vi "New Event Handler.vi"() -> ()   [LabVIEW 2010]
doc: "이 LLB에서 이 VI를 Old Event Handler.vi와 비교합니다. 이 VI는 폴링을 사용하는 대신 이벤트 구조를 사용하여 이벤트를 처리하는 방식을 결정합니다. 변환이 다른 케이스사이에서 동작하고 다른 이벤트사이에서 전달되는 데이터를 관리하는데 하나의 시프트 레지스터만을 사용하는 경우를 이해하는 것이 더 쉽습니다. 버튼을 클릭할 때를 결정하기 위해 사용자 인터페이스를 폴링하지 않습니다. 대신에 버튼을 클릭하거나 값 변경이 발생하기를 기다리고 발생한 이벤트에 따라 무슨 일을 수행할지 결정합니다.\n\n\"데이터 수집\":\n이 버튼을 클릭하면 데이터를 수집하는 케이스를 실행합니다. \n\n\"데이터 분석 및 제시\":\n이 버튼을 클릭하면 이전에 수집한 데이터를 분석합니다. 이 버튼을 클릭하기 전에는 어떤 데이터도 수집할 필요가 없습니다. 그러나 NULL 데이터셋에 대해 수행한 분석은 어떤 유용한 정보도 제공하지 않습니다.\n\n\"정지\":\n이 버튼을 클릭하면 VI 실행을 정지합니다."
panel:
  in  "새 버튼":bool
  in  "시간 웨이브폼":waveform(dbl)={"t0"=timestamp(0 s since 1904-01-01), "dt"=0.0, "Y"=[]}
  in  "정지":bool
  in  "분석":bool
  in  "수집":bool
  # "이 VI를 실행한 후, 버튼을 눌러 해당\n이벤트를 활성화하십시오. 완료시 정지 버튼을 누르십시오."
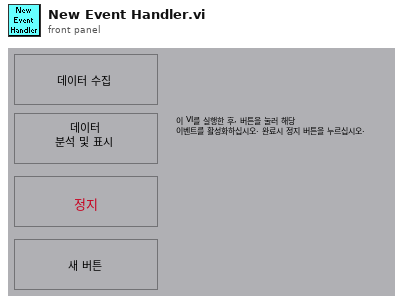
[diagram p1: front panel]
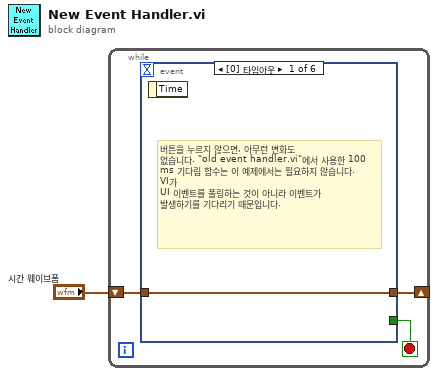
[diagram p0: block diagram]
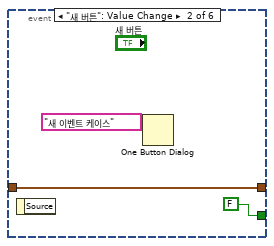
[diagram p2: hidden frame]
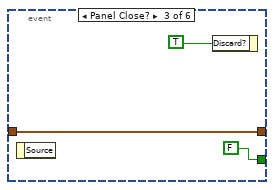
[diagram p3: hidden frame]
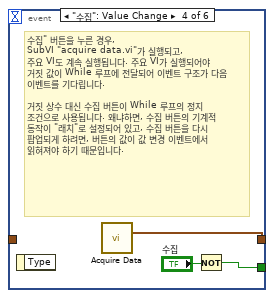
[diagram p4: hidden frame]
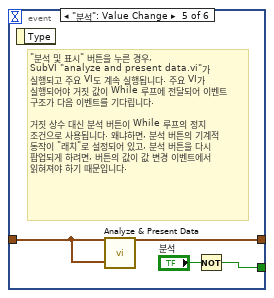
[diagram p5: hidden frame]
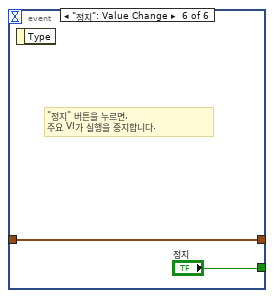
[diagram p6: hidden frame]
diagram:
  n1 = while {
    shift-right: [w4] -> _
    shift-left: "시간 웨이브폼" -> [w3]
    stop <- w2 stop-if-true
    n2 = event shown="[0] 타임아웃" {
      selector: _ -> [_ _ _ _ _ _]
      dyn-events: _ -> [_ _ _ _ _ _]
      timeout: _ -> [_ _ _ _ _ _]
      tunnel: [w5 w8 w10 w14 w17 w19] -> w4
      tunnel: w3 -> [w5 w8 w10 _ w17 w19]
      tunnel: [_ FALSE ("Stop") FALSE ("Stop") w12 w15 "정지"] -> w2
      event Timeout {
        # "버튼을 누르지 않으면, 아무런 변화도 \n없습니다. \"old event handler.vi\"에서 사용한 100 ms 기다림 함수는 이 예제에서는 필요하지 않습니다. VI가\nUI 이벤트를 폴링하는 것이 아니라 이벤트가 발생하기를 기다리기 때문입니다."
        n3 = event-data() -> ()  [unwired: 1 in, 1 out]
      }
      event "새 버튼": Value Change {
        n4 = event-data() -> ()  [unwired: 1 in, 1 out]
        n5 = One Button Dialog(message="새 이벤트 케이스") -> ()  [unwired: 1 in, 1 out]
      }
      event Panel Close? {
        n6 = event-data() -> ()  [unwired: 1 in, 1 out]
        n7 = event-data("Discard?"=TRUE) -> ()  [unwired: 1 in, 1 out]
      }
      event "수집": Value Change {
        # "수집\" 버튼을 누른 경우, \nSubVI \"acquire data.vi\"가 실행되고,\n주요 VI도 계속 실행됩니다. 주요 VI가 실행되어야 거짓 값이 While 루프에 전달되어 이벤트 구조가 다음 이벤트를 기다립니다.\n\n거짓 상수 대신 수집 버튼이 While 루프의 정지 조건으로 사용됩니다. 왜냐하면, 수집 버튼의 기계적 동작이 \"래치\"로 설정되어 있고, 수집 버튼을 다시 팝업되게 하려면, 버튼의 값이 값 변경 이벤트에서 읽혀져야 하기 때문입니다."
        n8 = event-data() -> ()  [unwired: 1 in, 1 out]
        n9 = call "Acquire Data.vi"() -> ("시간 웨이브폼"=w14:waveform(dbl))  [unwired: 2 in]
        n10 = Not(x="수집") -> (.not. x?=w12:bool)
      }
      event "분석": Value Change {
        # "\"분석 및 표시\" 버튼을 누른 경우,\nSubVI \"analyze and present data.vi\"가 실행되고 주요 VI도 계속 실행됩니다. 주요 VI가 실행되어야 거짓 값이 While 루프에 전달되어 이벤트 구조가 다음 이벤트를 기다립니다.\n\n거짓 상수 대신 분석 버튼이 While 루프의 정지 조건으로 사용됩니다. 왜냐하면, 분석 버튼의 기계적 동작이 \"래치\"로 설정되어 있고, 분석 버튼을 다시 팝업되게 하려면, 버튼의 값이 값 변경 이벤트에서 읽혀져야 하기 때문입니다."
        n11 = event-data() -> ()  [unwired: 1 in, 1 out]
        n12 = call "Analyze & Present Data.vi"("데이터"=w17) -> ()  [unwired: 2 in]
        n13 = Not(x="분석") -> (.not. x?=w15:bool)
      }
      event "정지": Value Change {
        # "\"정지\" 버튼을 누르면,\n주요 VI가 실행을 중지합니다."
        n14 = event-data() -> ()  [unwired: 1 in, 1 out]
      }
    }
  }
